vi "kinesis.vi"(8 "error in (no error)":errorcluster) -> (0 "error out":errorcluster, 1 "Z-Position":dbl, 2 "Y-Position":dbl, 3 "X-Position":dbl)   [LabVIEW 2016]
uses:
  C:/Users/Public/LabVIEW/BeamScanner/kinesis/Thorlabs.MotionControl.Controls.dll
  Thorlabs.MotionControl.Controls.dll
  C:/Users/Public/LabVIEW/BeamScanner/kinesis/Thorlabs.MotionControl.Benchtop.BrushlessMotorCLI.dll
  Thorlabs.MotionControl.Benchtop.BrushlessMotorCLI.dll
  C:/Users/Public/LabVIEW/BeamScanner/kinesis/Thorlabs.MotionControl.Benchtop.PiezoCLI.dll
  Thorlabs.MotionControl.Benchtop.PiezoCLI.dll
  C:/Users/Public/LabVIEW/BeamScanner/kinesis/Thorlabs.MotionControl.GenericPiezoCLI.dll
  Thorlabs.MotionControl.GenericPiezoCLI.dll
  resources/MotorPosition.vi
panel:
  in  "stop":bool
  in  "Z-Axis":refnum<k24>(container)
  in  "Y-Axis":refnum<k24>(container)
  in  "X-Axis":refnum<k24>(container)
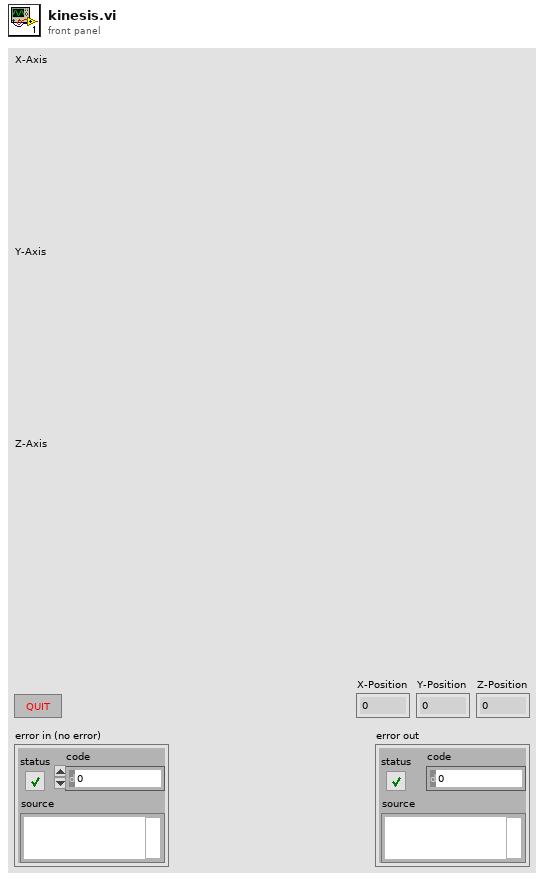
[diagram p1: front panel]
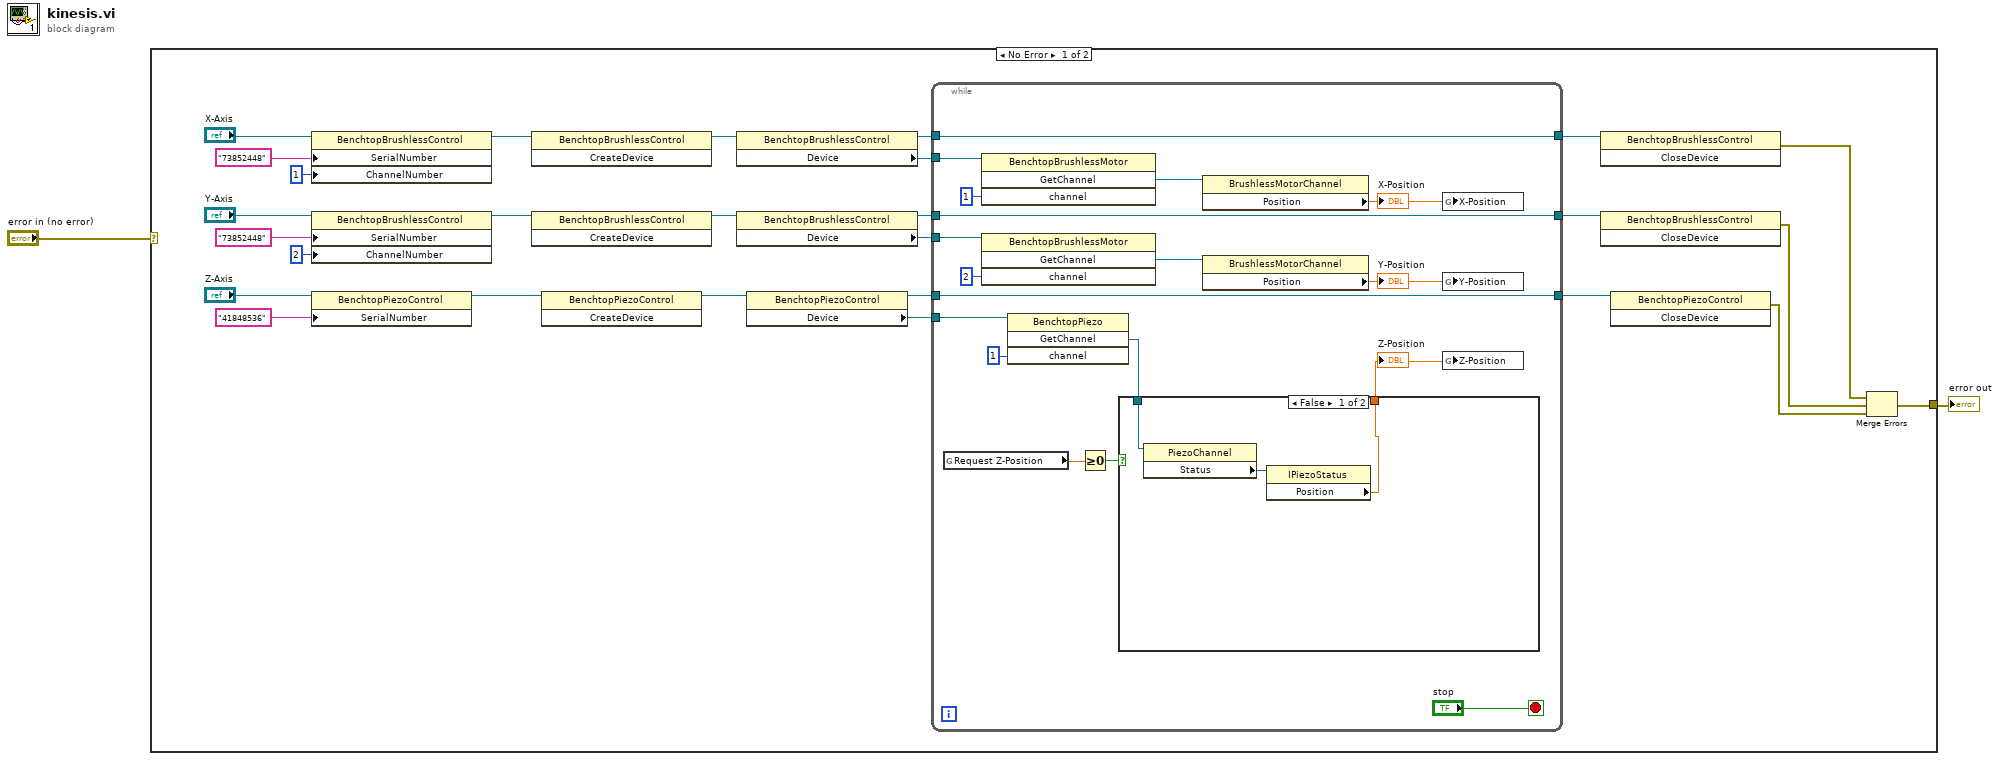
[diagram p0: block diagram]
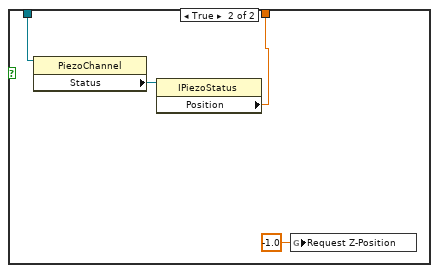
[diagram p2: hidden frame]
diagram:
  n1 = case shown="No Error" "error in (no error)" {
    selector: "error in (no error)" -> [_ w55]
    tunnel: [w7 w55] -> w1
    frame No Error {
      n2 = property class="BenchtopBrushlessControl"(reference="X-Axis", "SerialNumber"="73852448", "ChannelNumber"=1) -> (reference out=w24:refnum<k24>)  [unwired: 1 in, 1 out]
      n3 = property class="BenchtopBrushlessControl"(reference="Y-Axis", "SerialNumber"="73852448", "ChannelNumber"=2) -> (reference out=w23:refnum<k24>)  [unwired: 1 in, 1 out]
      n4 = property class="BenchtopPiezoControl"(reference="Z-Axis", "SerialNumber"="41848536") -> (reference out=w8:refnum<k24>)  [unwired: 1 in, 1 out]
      n5 = invoke class="BenchtopBrushlessControl" method="CreateDevice"(reference=w24) -> (reference out=w17:refnum<k24>)  [unwired: 2 in, 2 out]
      n6 = invoke class="BenchtopBrushlessControl" method="CreateDevice"(reference=w23) -> (reference out=w11:refnum<k24>)  [unwired: 2 in, 2 out]
      n7 = invoke class="BenchtopPiezoControl" method="CreateDevice"(reference=w8) -> (reference out=w14:refnum<k24>)  [unwired: 2 in, 2 out]
      n8 = property class="BenchtopBrushlessControl"(reference=w17) -> (reference out=w16:refnum<k24>, "Device"=w15:refnum<k24>)  [unwired: 1 in, 1 out]
      n9 = property class="BenchtopBrushlessControl"(reference=w11) -> (reference out=w10:refnum<k24>, "Device"=w9:refnum<k24>)  [unwired: 1 in, 1 out]
      n10 = property class="BenchtopPiezoControl"(reference=w14) -> (reference out=w13:refnum<k24>, "Device"=w12:refnum<k24>)  [unwired: 1 in, 1 out]
      n11 = while {
        tunnel: w16 -> [w47]
        tunnel: [w47] -> w22
        tunnel: [w46] -> w21
        tunnel: w10 -> [w46]
        tunnel: [w45] -> w20
        tunnel: w13 -> [w45]
        tunnel: w15 -> [w44]
        tunnel: w12 -> [w43]
        tunnel: w9 -> [w42]
        stop <- "stop" stop-if-true
        n12 = global read "MotorPosition.vi" "Request Z-Position"() -> (w33:dbl)
        n13 = invoke class="BenchtopBrushlessMotor" method="GetChannel"(reference=w44, "channel"=i16 1) -> ("GetChannel"=w41:refnum<k24>)  [unwired: 2 in, 3 out]
        n14 = invoke class="BenchtopBrushlessMotor" method="GetChannel"(reference=w42, "channel"=i16 2) -> ("GetChannel"=w37:refnum<k24>)  [unwired: 2 in, 3 out]
        n15 = invoke class="BenchtopPiezo" method="GetChannel"(reference=w43, "channel"=i16 1) -> ("GetChannel"=w30:refnum<k24>)  [unwired: 2 in, 3 out]
        n16 = Greater Or Equal To 0?(x=w33) -> (x >= 0?=w32:bool)
        n17 = case shown="False" w32 {
          tunnel: w30 -> [w49 w53]
          tunnel: [w48 w51] -> w31
          frame False {
            n18 = property class="PiezoChannel"(reference=w49) -> ("Status"=w50:refnum<k24>)  [unwired: 1 in, 2 out]
            n19 = property class="IPiezoStatus"(reference=w50) -> ("Position"=w48:dbl)  [unwired: 1 in, 2 out]
          }
          frame True {
            n20 = property class="PiezoChannel"(reference=w53) -> ("Status"=w52:refnum<k24>)  [unwired: 1 in, 2 out]
            n21 = property class="IPiezoStatus"(reference=w52) -> ("Position"=w51:dbl)  [unwired: 1 in, 2 out]
            n22 = global write "MotorPosition.vi" "Request Z-Position"(-1.0 ("Request Z-Position")) -> ()
          }
        }
        "Z-Position" <- w31
        n23 = property class="BrushlessMotorChannel"(reference=w41) -> ("Position"=w36:dbl)  [unwired: 1 in, 2 out]
        "X-Position" <- w36
        n24 = property class="BrushlessMotorChannel"(reference=w37) -> ("Position"=w35:dbl)  [unwired: 1 in, 2 out]
        "Y-Position" <- w35
        n25 = global write "MotorPosition.vi" "X-Position"(w36) -> ()
        n26 = global write "MotorPosition.vi" "Y-Position"(w35) -> ()
        n27 = global write "MotorPosition.vi" "Z-Position"(w31) -> ()
      }
      n28 = invoke class="BenchtopBrushlessControl" method="CloseDevice"(reference=w22) -> (error out=w4:errorcluster)  [unwired: 2 in, 2 out]
      n29 = invoke class="BenchtopBrushlessControl" method="CloseDevice"(reference=w21) -> (error out=w5:errorcluster)  [unwired: 2 in, 2 out]
      n30 = invoke class="BenchtopPiezoControl" method="CloseDevice"(reference=w20) -> (error out=w6:errorcluster)  [unwired: 2 in, 2 out]
      n31 = Merge Errors(w4, w5, w6) -> (w7:errorcluster)
    }
    frame Error {
    }
  }
  "error out" <- w1
